vi "SetClassQueueMessage.vi"(6 "QMessage":string, 8 "ErrorIn(No Error)":errorcluster caption="entrée d'erreur (pas d'erreur)", 9 "Data":variant, 10 "Menu déroulant":T1 items=["UpdateClassData", "UpdateMainClass", "UpdateDataBind", "ReInitDevice", "Custom", "ClosePan"], 11 "BaseDevice.lvclass":refnum<class "BaseDevice.lvclass">) -> (0 "sortie d'erreur":errorcluster, 3 "BaseDevice.lvclass Out":refnum<class "BaseDevice.lvclass">)   [LabVIEW 2019, in "BaseDevice.lvclass"]
uses:
  BaseDevice.lvclass
  ClassQueueMess.ctl
  BaseDevice.lvclass/BaseDevice.ctl
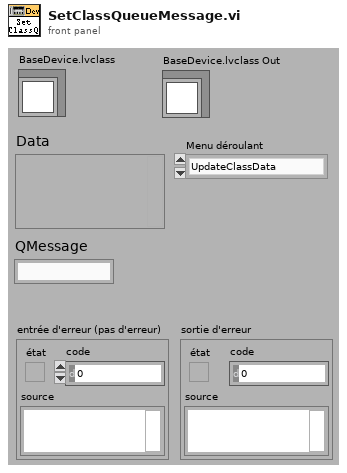
[diagram p1: front panel]
types:
  T1 = typedef "ClassQueueMess.ctl" = u16
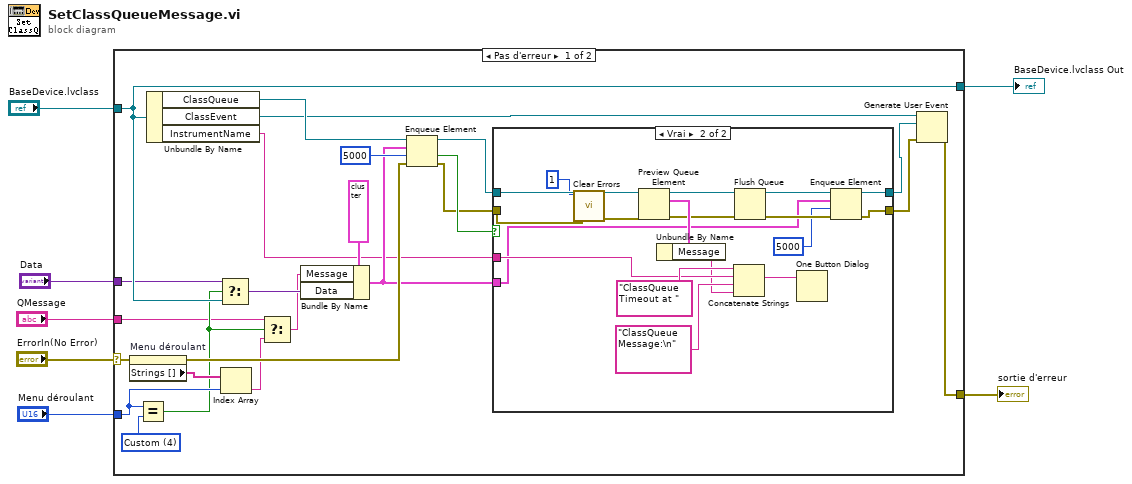
[diagram p0: block diagram]
diagram:
  n1 = case shown="Pas d'erreur" "ErrorIn(No Error)" {
    selector: "ErrorIn(No Error)" -> [w28 w53]
    tunnel: [w24 w53] -> w7
    tunnel: "BaseDevice.lvclass" -> [w14 w52]
    tunnel: [w14 w52] -> w4
    tunnel: "Menu déroulant" -> [w16 _]
    tunnel: "Data" -> [w13 _]
    tunnel: "QMessage" -> [w8 _]
    frame No Error {
      w15 = T1 4 items=["UpdateClassData", "UpdateMainClass", "UpdateDataBind", "ReInitDevice", "Custom", "ClosePan"] ("Menu déroulant")
      n2 = property on="Menu déroulant" class="MDér (strict)"(error in=w28) -> (error out=w25:errorcluster, "Strings []"=w27:string[])  [unwired: 1 in, 1 out]
      n3 = Equal?(x=w16, y=w15) -> (x = y?=w9:bool)
      n4 = Unbundle By Name(w14) -> ("ClassQueue"=w31:refnum<queue>, "ClassEvent"=w30:refnum<user-event>, "InstrumentName"=w19:string)
      n5 = Select(t=w13, s=w9, f=w14) -> (s? t:f=w12:variant)
      n6 = Index Array(array=w27, index=w16) -> (element=w11:string)
      n7 = Select(t=w8, s=w9, f=w11) -> (s? t:f=w10:string)
      n8 = Bundle By Name(cluster=cluster{"Message":string, "Data":variant, i32} {"Message"="", "Data"=variant, 0} ("élément"), "Message"=w10, "Data"=w12) -> (w20:cluster{"Message":string, "Data":variant, i32})
      n9 = Enqueue Element(queue=w31, element=w20, timeout in ms (-1)=5000 ("timeout en ms (-1)"), error in (no error)=w25) -> (queue out=w22:refnum<queue>, timed out?=w23:bool, error out=w21:errorcluster)
      n10 = case shown="Vrai" w23 {
        tunnel: w22 -> [w32 w51]
        tunnel: w21 -> [w33 w36]
        tunnel: w20 -> [_ w40]
        tunnel: w19 -> [_ w47]
        tunnel: [w33 w39] -> w18
        tunnel: [w32 w37] -> w17
        frame False {
        }
        frame True {
          n11 = call <vilib>:"Clear Errors.vi"("error in (no error)"=w36, "specific error code to clear (0: all)"=1) -> ("error out"=w35:errorcluster)  [unwired: 4 in, 1 out]
          n12 = Preview Queue Element(queue=w51, error in (no error)=w35) -> (queue out=w44:refnum<queue>, element=w50:cluster{"Message":string, "Data":variant, i32}, error out=w42:errorcluster)  [unwired: 1 in, 1 out]
          n13 = Unbundle By Name(w50) -> ("Message"=w45:string)
          n14 = Concatenate Strings("ClassQueue Timeout at " ("chaîne"), w47, "ClassQueue Message:\n" ("chaîne"), w45) -> (w49:string)
          n15 = Flush Queue(queue=w44, error in (no error)=w42) -> (queue out=w43:refnum<queue>, error out=w41:errorcluster)  [unwired: 1 out]
          n16 = One Button Dialog(message=w49) -> ()  [unwired: 1 in, 1 out]
          n17 = Enqueue Element(queue=w43, element=w40, timeout in ms (-1)=5000 ("timeout en ms (-1)"), error in (no error)=w41) -> (queue out=w37:refnum<queue>, error out=w39:errorcluster)  [unwired: 1 out]
        }
      }
      n18 = Generate User Event(user event=w30, event data cluster=w17, error in=w18) -> (error out=w24:errorcluster)  [unwired: 1 in, 1 out]
    }
    frame Error {
    }
  }
  "sortie d'erreur" <- w7
  "BaseDevice.lvclass Out" <- w4
